vi "Relative_path_defi.vi"(10 "Equip list":string[](array[string]), 11 "path":path) -> (1 "Path string":string[](array[string]), 2 "Array":string[](array[string]), 3 "Relative Path":path[](array[path]))   [LabVIEW 2024, in "Launcher_DTU.lvlib"]
uses:
  Launcher_DTU.lvlib
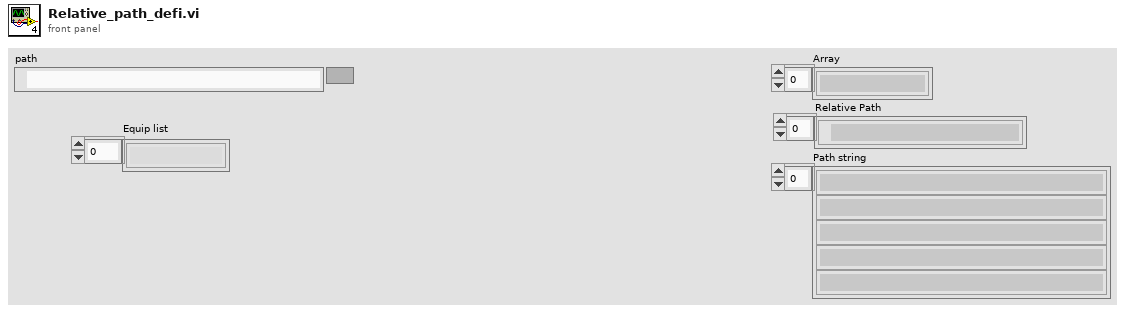
[diagram p1: front panel]
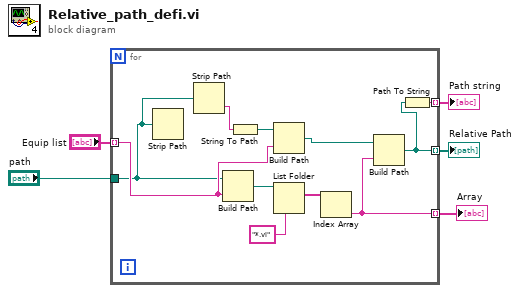
[diagram p0: block diagram]
diagram:
  n1 = for {
    tunnel: "path" -> [w6]
    tunnel: "Equip list" -> [w11] mode=indexing
    tunnel: [w14] -> w4 mode=indexing
    tunnel: [w9] -> w3 mode=indexing
    tunnel: [w8] -> w2 mode=indexing
    n2 = Strip Path(path=w6) -> ()  [unwired: 2 out]
    n3 = Strip Path(path=w6) -> (name=w7:string)  [unwired: 1 out]
    n4 = Build Path(base path=w6, name or relative path=w11) -> (appended path=w13:path)
    n5 = String To Path(string=w7) -> (path=w12:path)
    n6 = Build Path(base path=w12, name or relative path=w11) -> (appended path=w10:path)
    n7 = List Folder(path=w13, pattern="*.vi") -> (filenames=w15:string[])  [unwired: 2 in, 3 out]
    n8 = Index Array(array=w15) -> (element=w14:string)  [unwired: 1 in]
    n9 = Build Path(base path=w10, name or relative path=w14) -> (appended path=w9:path)
    n10 = Path To String(path=w9) -> (string=w8:string)
  }
  "Array" <- w4
  "Relative Path" <- w3
  "Path string" <- w2
